vi "Nattify - Get FP Objects Arrangement Info.vi"(0 "VI reference":refnum<vi>, 11 "error in":errorcluster) -> (4 "FP objects arrangement info":T1, 15 "error out":errorcluster)   [LabVIEW 2020]
uses:
  Nattify - FP Objects Arrangement Info.ctl
  <resource>/dialog/lvconfig.llb/LV Config Read Numeric (I32).vi
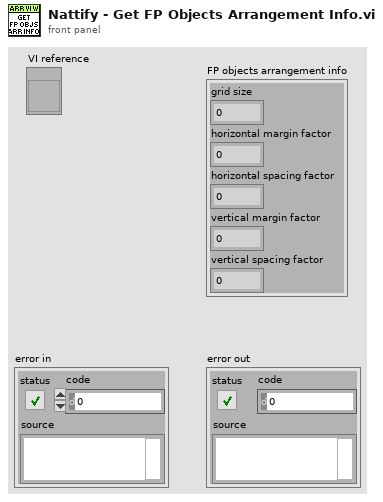
[diagram p1: front panel]
types:
  T1 = typedef "Nattify - FP Objects Arrangement Info.ctl" = cluster{"grid size":i32, "horizontal margin factor":i32, "horizontal spacing factor":i32, "vertical margin factor":i32, "vertical spacing factor":i32}
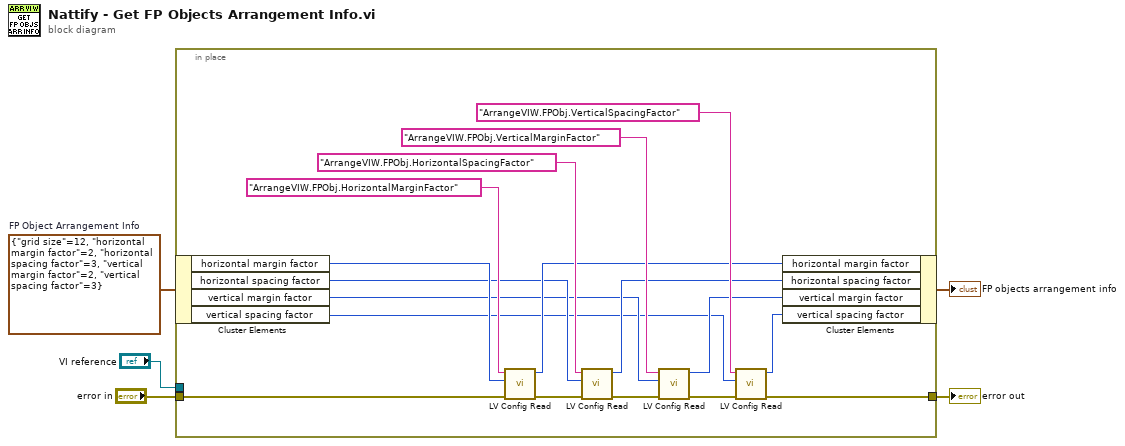
[diagram p0: block diagram]
diagram:
  w3 = T1 {"grid size"=12, "horizontal margin factor"=2, "horizontal spacing factor"=3, "vertical margin factor"=2, "vertical spacing factor"=3}  # FP Object Arrangement Info
  n1 = in-place {
    in-place-border: "error in" -> [w14]
    in-place-border: [w15] -> w4
    in-place-border: "VI reference" -> [_]
    n2 = in-place-cluster #1(w3) -> ("horizontal margin factor"=w9:i32, "horizontal spacing factor"=w8:i32, "vertical margin factor"=w7:i32, "vertical spacing factor"=w6:i32)
    n3 = call-poly <resource>:"LV Config Read.vi"("error in"=w14, "default value"=w9, "key"="ArrangeVIW.FPObj.HorizontalMarginFactor") -> ("error out"=w18:errorcluster, "value"=w13:i32)  [unwired: 2 in, 1 out]
    n4 = call-poly <resource>:"LV Config Read.vi"("error in"=w18, "default value"=w8, "key"="ArrangeVIW.FPObj.HorizontalSpacingFactor") -> ("error out"=w17:errorcluster, "value"=w12:i32)  [unwired: 2 in, 1 out]
    n5 = call-poly <resource>:"LV Config Read.vi"("error in"=w17, "default value"=w7, "key"="ArrangeVIW.FPObj.VerticalMarginFactor") -> ("error out"=w16:errorcluster, "value"=w11:i32)  [unwired: 2 in, 1 out]
    n6 = call-poly <resource>:"LV Config Read.vi"("error in"=w16, "default value"=w6, "key"="ArrangeVIW.FPObj.VerticalSpacingFactor") -> ("error out"=w15:errorcluster, "value"=w10:i32)  [unwired: 2 in, 1 out]
    n7 = in-place-cluster #1("horizontal margin factor"=w13, "horizontal spacing factor"=w12, "vertical margin factor"=w11, "vertical spacing factor"=w10) -> (→"FP objects arrangement info":T1)
  }
  "error out" <- w4
